vi "CAN write.vi"(4 "error in (no error)":errorcluster, 5 "Data":u8[](array[numeric]), 6 "COB id":i32, 7 "CANopen in":refnum<class "CANopen.lvclass">) -> (0 "error out":errorcluster, 3 "CANopen out":refnum<class "CANopen.lvclass">)   [LabVIEW 2017, in "canopen.lvlib" / "CANopen.lvclass"]
doc: "Sends a bunch of data to a specific COB-ID."
uses:
  CANopen.lvclass
  CANopen.lvclass/CANopen.ctl
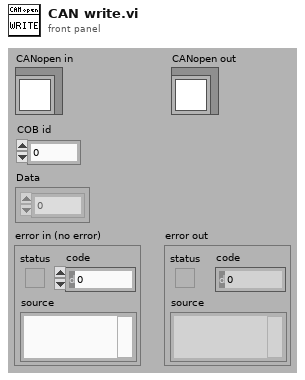
[diagram p1: front panel]
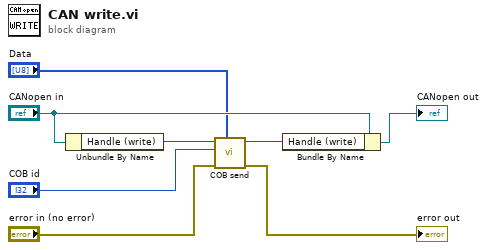
[diagram p0: block diagram]
diagram:
  n1 = Unbundle By Name("CANopen in") -> ("Handle (write)"=w6:i32)
  n2 = call "COB send.vi"("Data"="Data", "error in (no error)"="error in (no error)", "COB id"="COB id", "Handle in"=w6) -> ("error out"=→"error out":errorcluster, "Handle out"=w5:i32)  [unwired: 1 in, 2 out]
  n3 = Bundle By Name(cluster="CANopen in", "Handle (write)"=w5) -> (→"CANopen out":refnum<class "CANopen.lvclass">)
